vi "Obtain New Credit and cambio from UI.vi"(8 "error in (no error)":errorcluster, 9 "Cambio":i32, 10 "Credito":i32, 11 "Dinero in":refnum<class "Dinero.lvclass">) -> (0 "error out":errorcluster, 3 "Dinero out":refnum<class "Dinero.lvclass">)   [LabVIEW 2020, in "Dinero.lvlib" / "Dinero.lvclass"]
uses:
  Dinero.lvclass
  Dinero.lvclass/Dinero.ctl
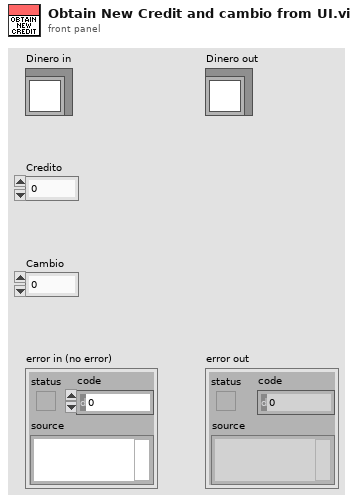
[diagram p1: front panel]
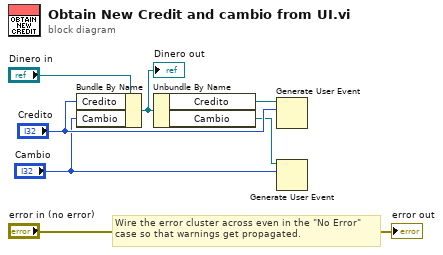
[diagram p0: block diagram]
diagram:
  # "Wire the error cluster across even in the \"No Error\"\ncase so that warnings get propagated."
  n1 = Bundle By Name(cluster="Dinero in", "Credito"="Credito", "Cambio"="Cambio") -> (w5:refnum<class "Dinero.lvclass">)
  "Dinero out" <- w5
  n2 = Unbundle By Name(w5) -> ("Credito"=w4:refnum<user-event>, "Cambio"=w2:refnum<user-event>)
  n3 = Generate User Event(user event=w4, event data cluster="Credito") -> ()  [unwired: 2 in, 2 out]
  n4 = Generate User Event(user event=w2, event data cluster="Cambio") -> ()  [unwired: 2 in, 2 out]
  "error out" <- "error in (no error)"
